vi "Thermocouple Read.vi"() -> (0 "Cluster":T1 {"Resevoir Temp" format="%.1g"; "Inlet Dry Bulb Temp" format="%.1g"; "Inlet Wet Bulb Temp" format="%.1g"; "Outlet Wet Bulb Temp" format="%.1g"; "Outlet Dry Bulb Temp" format="%.1g"; "Inlet Water Temp" format="%.1g"; "Outlet Water Temp" format="%.1g"})   [LabVIEW 2012]
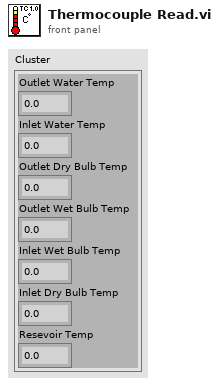
[diagram p1: front panel]
types:
  T1 = cluster{"Outlet Water Temp":dbl, "Inlet Water Temp":dbl, "Outlet Dry Bulb Temp":dbl, "Outlet Wet Bulb Temp":dbl, "Inlet Wet Bulb Temp":dbl, "Inlet Dry Bulb Temp ":dbl, "Resevoir Temp":dbl}
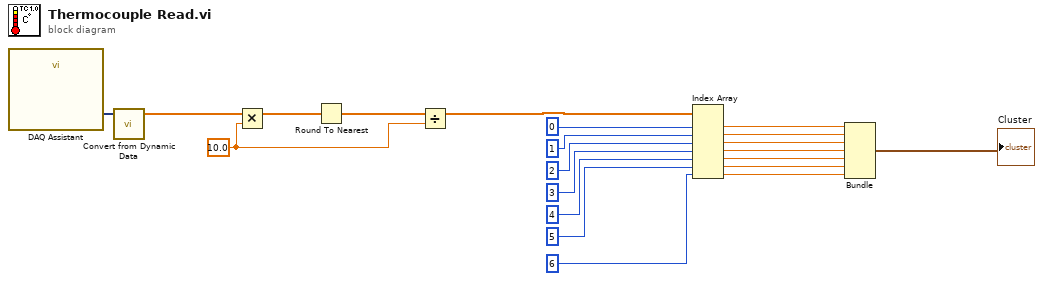
[diagram p0: block diagram]
diagram:
  w1 = sgl 10.0
  n1 = call "DAQ Assistant"() -> ("data"=w21:dynamicdata)  [unwired: 17 in, 2 out]
  n2 = call "Convert from Dynamic Data"("Dynamic Data Type"=w21) -> ("Array"=w20:dbl[])  [unwired: 3 in]
  n3 = Multiply(x=w20, y=w1) -> (x*y=w4:dbl[])
  n4 = Round To Nearest(number=w4) -> (nearest integer value=w3:dbl[])
  n5 = Divide(x=w3, y=w1) -> (x/y=w2:dbl[])
  n6 = Index Array(array=w2, index #1=0, index #2=1, index #3=2, index #4=3, index #5=4, index #6=5, index #7=6) -> (element #1=w13:dbl, element #2=w12:dbl, element #3=w11:dbl, element #4=w10:dbl, element #5=w9:dbl, element #6=w8:dbl, element #7=w6:dbl)
  n7 = Bundle(w13, w12, w11, w10, w9, w8, w6) -> (→"Cluster":cluster{dbl, dbl, dbl, dbl, dbl, dbl, dbl})  [unwired: 1 in]
